vi "Configure.vi"(7 "Setpoint Deceleration":u32, 8 "error in (no error)":errorcluster, 9 "Setpoint Acceleration":u32, 10 "Setpoint Velocity":u32, 11 "IgusMotorDrive in":refnum<class "IgusMotorDrive.lvclass">) -> (0 "error out":errorcluster, 3 "IgusMotorDrive out":refnum<class "IgusMotorDrive.lvclass">)   [LabVIEW 2016, in "IgusMotorDrive.lvclass"]
uses:
  IgusMotorDrive.lvclass
  motor-drive/MotorDrive.lvclass
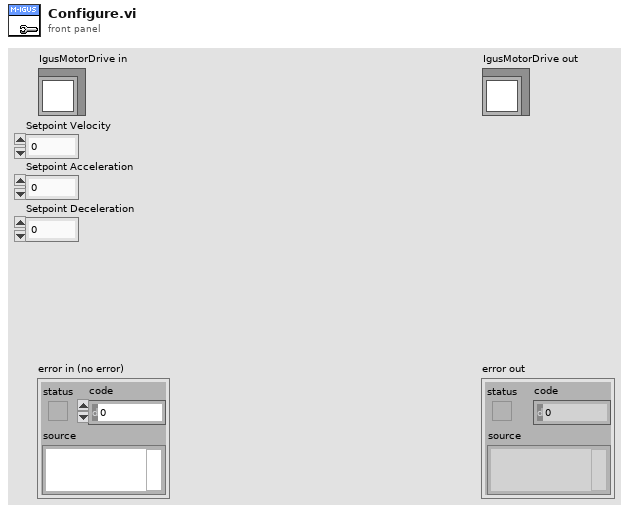
[diagram p1: front panel]
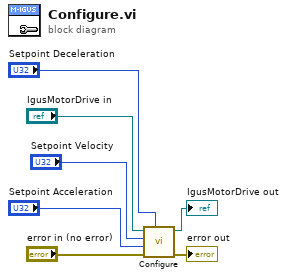
[diagram p0: block diagram]
diagram:
  n1 = call-parent "Configure.vi"("Setpoint Deceleration"="Setpoint Deceleration", "error in (no error)"="error in (no error)", "Setpoint Acceleration"="Setpoint Acceleration", "Setpoint Velocity"="Setpoint Velocity", "MotorDrive in"="IgusMotorDrive in") -> ("error out"=→"error out":errorcluster, "MotorDrive out"=→"IgusMotorDrive out":refnum<class "IgusMotorDrive.lvclass">)  [unwired: 5 in]
